vi "SwerveMapping.vi"() -> ()   [LabVIEW 2018]
panel:
  out "FrontLeftDriveOut":dbl
  out "FrontRightDriveOut":dbl
  out "RearLeftDriveOut":dbl
  out "RearRightDriveOut":dbl
  in  "RearRightDriveIn":dbl
  in  "RearLeftDriveIn":dbl
  in  "FrontRightDriveIn":dbl
  in  "FrontLeftDriveIn":dbl
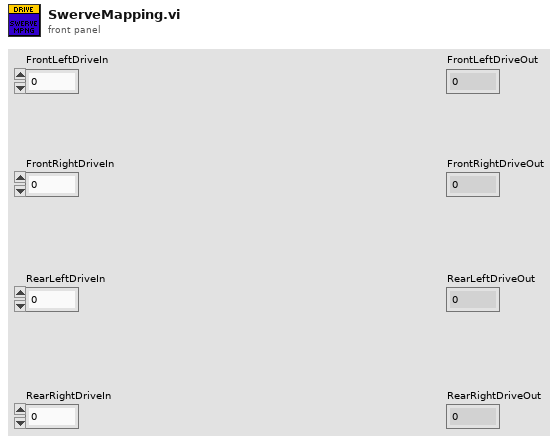
[diagram p1: front panel]
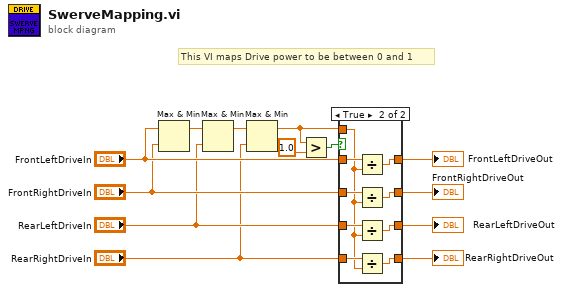
[diagram p0: block diagram]
diagram:
  # "This VI maps Drive power to be between 0 and 1"
  n1 = Max & Min(x="FrontLeftDriveIn", y="FrontRightDriveIn") -> (max(x,y)=w9:dbl)  [unwired: 1 out]
  n2 = Max & Min(x=w9, y="RearLeftDriveIn") -> (max(x,y)=w10:dbl)  [unwired: 1 out]
  n3 = Max & Min(x=w10, y="RearRightDriveIn") -> (max(x,y)=w11:dbl)  [unwired: 1 out]
  n4 = Greater?(x=w11, y=1.0) -> (0:w12:bool)
  n5 = case shown="True" w12 {
    tunnel: w11 -> [_ w22]
    tunnel: "FrontLeftDriveIn" -> [w17 w26]
    tunnel: "FrontRightDriveIn" -> [w16 w25]
    tunnel: "RearLeftDriveIn" -> [w15 w24]
    tunnel: "RearRightDriveIn" -> [w14 w23]
    tunnel: [w17 w21] -> w4
    tunnel: [w16 w20] -> w3
    tunnel: [w15 w19] -> w2
    tunnel: [w14 w18] -> w1
    frame False {
    }
    frame True {
      n6 = Divide(x=w26, y=w22) -> (x/y=w21:dbl)
      n7 = Divide(x=w25, y=w22) -> (x/y=w20:dbl)
      n8 = Divide(x=w24, y=w22) -> (x/y=w19:dbl)
      n9 = Divide(x=w23, y=w22) -> (x/y=w18:dbl)
    }
  }
  "FrontLeftDriveOut" <- w4
  "FrontRightDriveOut" <- w3
  "RearLeftDriveOut" <- w2
  "RearRightDriveOut" <- w1
